vi "Encoder_RegisterEachEncoder.vi"(2 "error in (no error)":errorcluster, 3 "RobotDrive refnum name":string="My RobotDrive RefNum", 4 "RobotEncoderRef":T5) -> (0 "error out":errorcluster, 1 "RobotEncoderRef out":T5)   [LabVIEW 2013]
uses:
  <vilib>/Rock Robotics/WPI/Encoder/WPI_EncoderDevRef.ctl
  <vilib>/Rock Robotics/SystemInterfaces/Encoder/FPGA_EncoderIdx.ctl
  <vilib>/Rock Robotics/SystemInterfaces/Counter/FPGA_CounterCtrSystemIndex.ctl
  <vilib>/Rock Robotics/WPI/Encoder/WPI_EncoderType.ctl
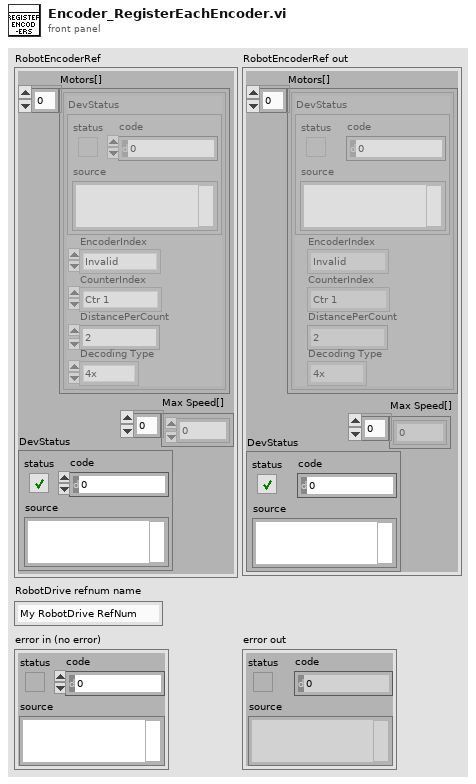
[diagram p1: front panel]
types:
  T1 = typedef "WPI_EncoderDevRef.ctl" = cluster{"DevStatus":errorcluster, "EncoderIndex":T2, "CounterIndex":T3, "DistancePerCount":dbl, "Decoding Type":T4}
  T2 = typedef "FPGA_EncoderIdx.ctl" = enum8{"Enc 0", "Enc 1", "Enc 2", "Enc 3", "Invalid"}
  T3 = typedef "FPGA_CounterCtrSystemIndex.ctl" = enum8{"Ctr 0", "Ctr 1", "Ctr 2", "Ctr 3", "Ctr 4", "Ctr 5", "Ctr 6", "Ctr 7", "Invalid"}
  T4 = typedef "WPI_EncoderType.ctl" = enum16{"1x", "2x", "4x"}
  T5 = cluster{"Motors[]":T1[], "DevStatus":errorcluster, "Max Speed[]":dbl[]}
  T6 = enum16{"Rear Left Motor", "Rear Right Motor", "Front Left Motor", "Front Right Motor"}
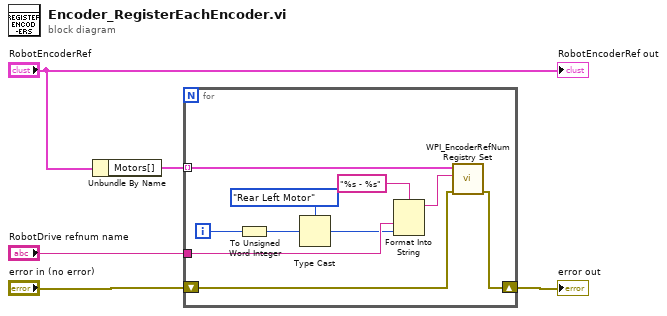
[diagram p0: block diagram]
diagram:
  n1 = Unbundle By Name("RobotEncoderRef") -> ("Motors[]"=w3:T1[])
  n2 = for {
    shift-right: [w14] -> w5
    shift-left: "error in (no error)" -> [w15]
    tunnel: w3 -> [w13] mode=indexing
    tunnel: "RobotDrive refnum name" -> [w11]
    i -> [w10]
    n3 = To Unsigned Word Integer(number=w10) -> (unsigned 16bit integer=w9:u16)
    n4 = Type Cast(type=T6."Rear Left Motor", x=w9) -> (*(type *) &x=w8:T6)
    n5 = Format Into String(format string="%s - %s", w11, w8) -> (resulting string=w12:string)  [unwired: 2 in, 1 out]
    n6 = call <vilib>:"WPI_EncoderRefNum Registry Set.vi"("error in (no error)"=w15, "refnum name"=w12, "EncoderDevRef"=w13) -> ("error out"=w14:errorcluster)  [unwired: 7 in, 1 out]
  }
  "error out" <- w5
  "RobotEncoderRef out" <- "RobotEncoderRef"
